vi "End.vi"(8 "error in (no error)":errorcluster, 11 "Channel Manager in":refnum<class "Channel Manager.lvclass">) -> (0 "error out":errorcluster, 3 "Channel Manager out":refnum<class "Channel Manager.lvclass">)   [LabVIEW 2018, in "Channel Manager.lvclass"]
uses:
  Channel Manager.lvclass
  Channel Manager.lvclass/Channel Manager.ctl
  Channel/Channel.lvclass
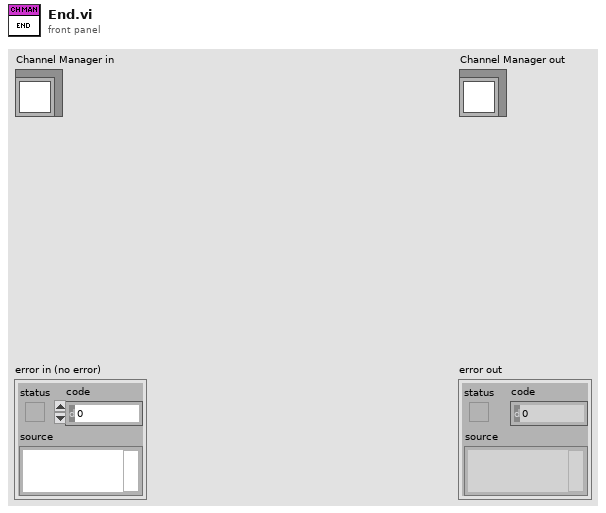
[diagram p1: front panel]
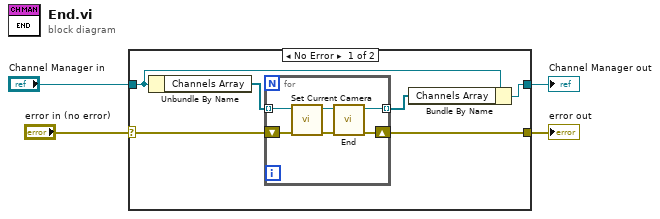
[diagram p0: block diagram]
diagram:
  n1 = case shown="No Error" "error in (no error)" {
    selector: "error in (no error)" -> [w8 w18]
    tunnel: [w7 w18] -> w3
    tunnel: [w9 w17] -> w1
    tunnel: "Channel Manager in" -> [w10 w17]
    frame No Error {
      n2 = Unbundle By Name(w10) -> ("Channels Array"=w6:refnum<class "Channel.lvclass">[])
      n3 = for {
        shift-right: [w15] -> w7
        shift-left: w8 -> [w12]
        tunnel: [w16] -> w5 mode=indexing
        tunnel: w6 -> [w11] mode=indexing
        n4 = call "Set Current Camera.vi"("error in (no error)"=w12, "Channel in"=w11) -> ("error out"=w13:errorcluster, "Channel out"=w14:refnum<class "Channel.lvclass">)  [unwired: 8 in]
        n5 = call "End.vi"("error in (no error)"=w13, "Channel in"=w14) -> ("error out"=w15:errorcluster, "Channel out"=w16:refnum<class "Channel.lvclass">)  [unwired: 8 in]
      }
      n6 = Bundle By Name(cluster=w10, "Channels Array"=w5) -> (w9:refnum<class "Channel Manager.lvclass">)
    }
    frame Error {
    }
  }
  "error out" <- w3
  "Channel Manager out" <- w1
